vi "Read U16.vi"(11 "unsigned byte array":u8[](array[numeric])) -> (3 "U16 Out":u16, 5 "rest of array":u8[](array[numeric]))   [LabVIEW 2015]
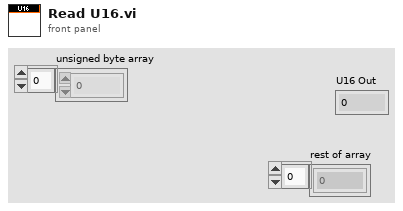
[diagram p1: front panel]
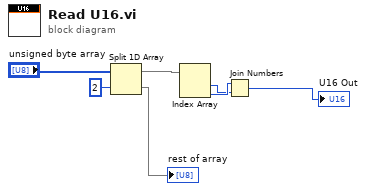
[diagram p0: block diagram]
diagram:
  n1 = Split 1D Array(array="unsigned byte array", index=2) -> (first subarray=w5:u8[], second subarray=→"rest of array":u8[])
  n2 = Index Array(array=w5) -> (element #1=w6:u8, element #2=w7:u8)  [unwired: 2 in]
  n3 = Join Numbers(hi=w7, lo=w6) -> ((hi.lo)=→"U16 Out":u16)
